vi "tcp esp32.vi"() -> ()   [LabVIEW 2020]
uses:
  <vilib>/ErrorRing/Error Ring.xnode
panel:
  in  "Boolean":bool
  in  "stop":bool
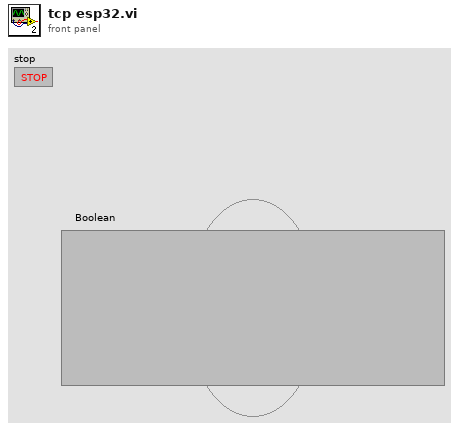
[diagram p1: front panel]
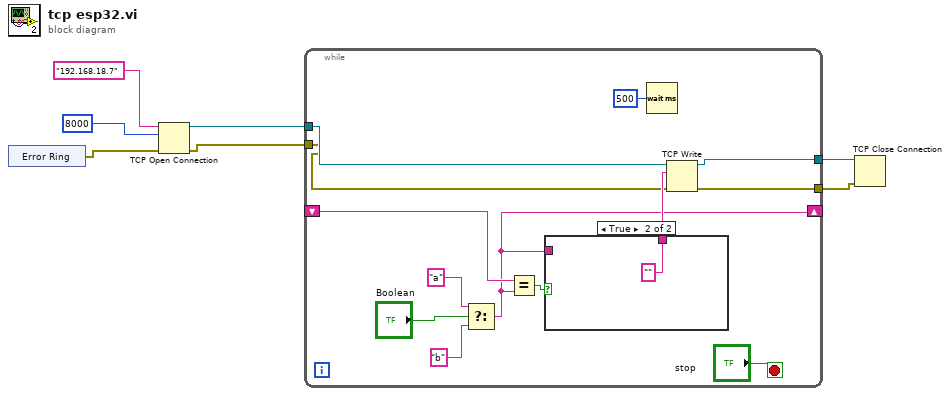
[diagram p0: block diagram]
diagram:
  n1 = xnode "Error Ring"() -> ("error out"=w1:errorcluster)
  n2 = TCP Open Connection(address="192.168.18.7", remote port or service name=u16 8000, error in (no error)=w1) -> (connection ID=w5:refnum<k5>, error out=w4:errorcluster)  [unwired: 2 in]
  n3 = while {
    tunnel: w5 -> [w12]
    tunnel: w4 -> [w11]
    shift-right: [w13] -> _
    shift-left: _ -> [w16]
    tunnel: [w10] -> w3
    tunnel: [w9] -> w2
    stop <- "stop" stop-if-true
    n4 = Select(t="a", s="Boolean", f="b") -> (s? t:f=w13:string)
    n5 = Equal?(x=w16, y=w13) -> (x = y?=w15:bool)
    n6 = case shown="True" w15 {
      tunnel: [w21 ""] -> w14
      tunnel: w13 -> [w21 _]
      frame False {
      }
      frame True {
      }
    }
    n7 = Wait (ms)(milliseconds to wait=u32 500) -> ()  [unwired: 1 out]
    n8 = TCP Write(connection ID=w12, data in=w14, error in (no error)=w11) -> (connection ID out=w10:refnum<k5>, error out=w9:errorcluster)  [unwired: 1 in, 1 out]
  }
  n9 = TCP Close Connection(connection ID=w3, error in (no error)=w2) -> ()  [unwired: 1 in, 2 out]
